vi "Check error type.vi"(8 "error in (no error)":errorcluster, 10 "Error cluster":T1={"jth object"="", "required object name"="", "Array element index"=0, "Element found?"=TRUE, "Array of clusters?"=FALSE, "key"="", "value"="", "key given?"=FALSE}, 11 "Datatype":T2) -> (0 "error out":errorcluster, 3 "Error string":string)   [LabVIEW 2015]
uses:
  Type Definitions/Basic datatypes.ctl
  Type Definitions/Error cluster.ctl
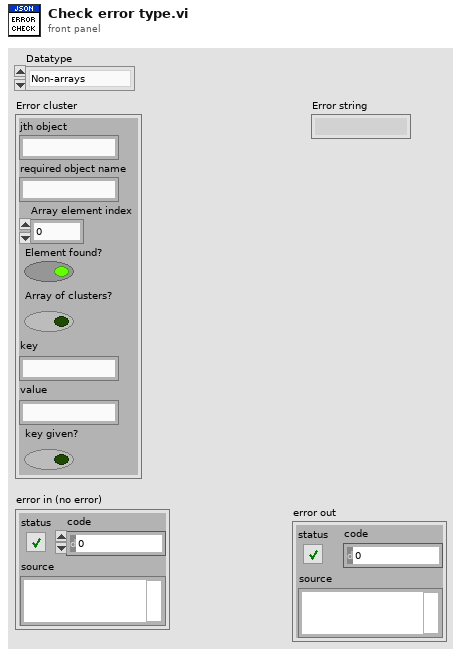
[diagram p1: front panel]
types:
  T1 = typedef "Error cluster.ctl" = cluster{"jth object":string, "required object name":string, "Array element index":u64, "Element found?":bool, "Array of clusters?":bool, "key":string, "value":string, "key given?":bool}
  T2 = typedef "Basic datatypes.ctl" = enum16{"Non-arrays", "Non-indexed array", "Indexed array"}
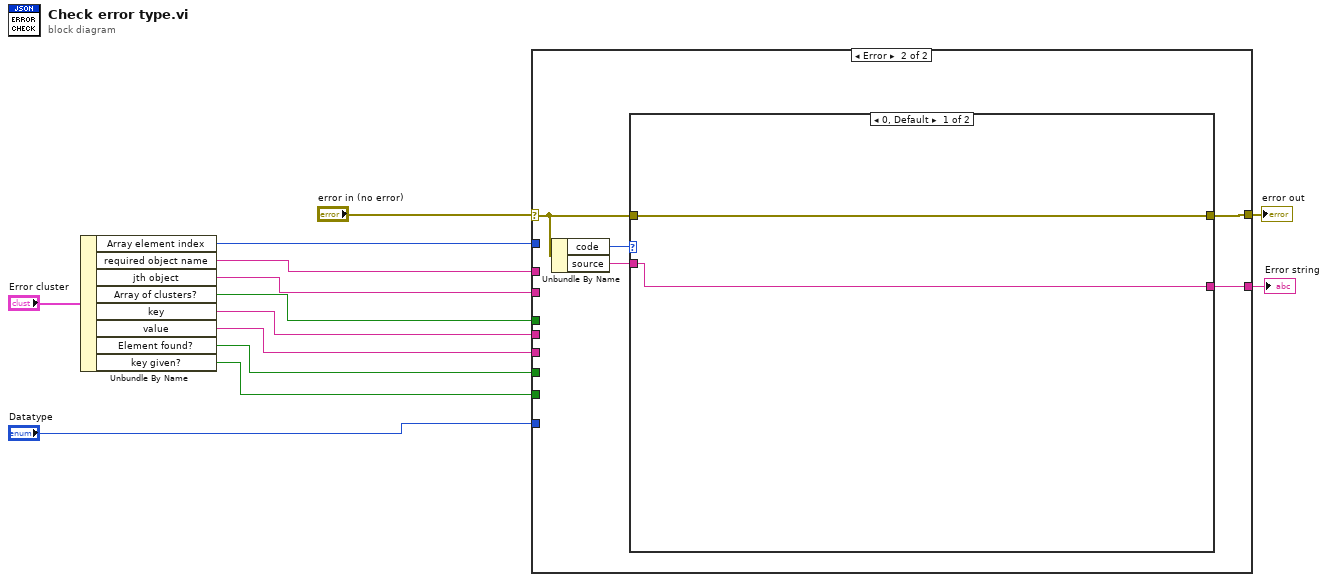
[diagram p0: block diagram]
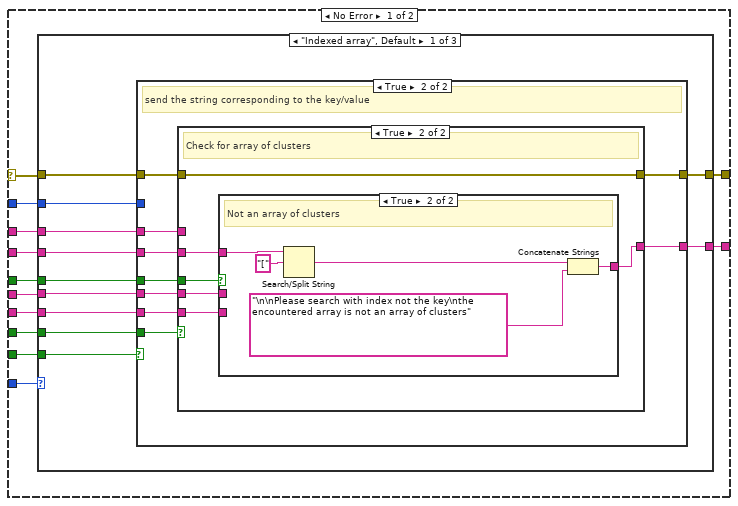
[diagram p2: hidden frame]
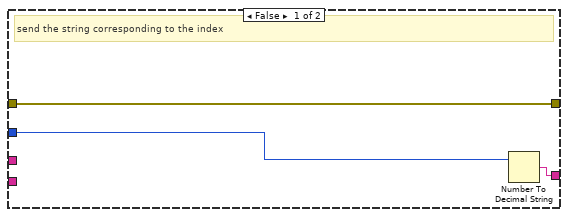
[diagram p3: hidden frame]
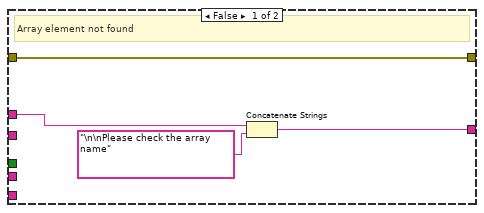
[diagram p4: hidden frame]
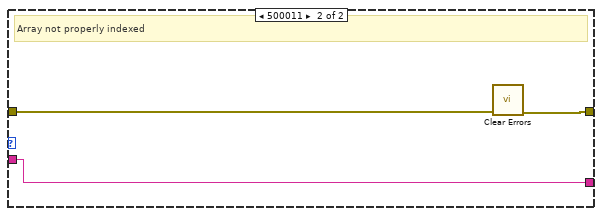
[diagram p8: hidden frame]
diagram:
  n1 = Unbundle By Name("Error cluster") -> ("Array element index"=w9:u64, "required object name"=w8:string, "jth object"=w7:string, "Array of clusters?"=w6:bool, "key"=w5:string, "value"=w4:string, "Element found?"=w2:bool, "key given?"=w3:bool)
  n2 = case shown="Error" "error in (no error)" {
    selector: "error in (no error)" -> [w14 w71]
    tunnel: [w25 w69] -> w13
    tunnel: [w24 w72] -> w12
    tunnel: "Datatype" -> [w23 _]
    tunnel: w9 -> [w22 _]
    tunnel: w8 -> [w21 _]
    tunnel: w7 -> [w20 _]
    tunnel: w6 -> [w19 _]
    tunnel: w5 -> [w18 _]
    tunnel: w4 -> [w17 _]
    tunnel: w3 -> [w16 _]
    tunnel: w2 -> [w15 _]
    frame No Error {
      n3 = case shown="\"Indexed array\", Default" w23 {
        tunnel: w21 -> [w26 _ w68]
        tunnel: w17 -> [w36 _ _]
        tunnel: w22 -> [w35 _ _]
        tunnel: w16 -> [w34 _ _]
        tunnel: w18 -> [w33 _ _]
        tunnel: [w32 w66 w68] -> w25
        tunnel: w20 -> [w31 w66 _]
        tunnel: w14 -> [w30 w65 w67]
        tunnel: [w29 w65 w67] -> w24
        tunnel: w15 -> [w28 _ _]
        tunnel: w19 -> [w27 _ _]
        frame "Indexed array", Default {
          n4 = case shown="True" w34 {
            tunnel: w33 -> [_ w46]
            tunnel: [w38 w47] -> w32
            tunnel: w35 -> [w39 _]
            tunnel: w36 -> [_ w48]
            tunnel: w26 -> [_ w44]
            tunnel: w31 -> [_ w45]
            tunnel: w30 -> [w37 w42]
            tunnel: [w37 w43] -> w29
            tunnel: w28 -> [_ w41]
            tunnel: w27 -> [_ w40]
            frame False {
              # "send the string corresponding to the index"
              n5 = Number To Decimal String(number=w39) -> (decimal integer string=w38:string)  [unwired: 1 in]
            }
            frame True {
              # "send the string corresponding to the key/value"
              n6 = case shown="True" w41 {
                tunnel: w48 -> [_ w58]
                tunnel: [w50 w57] -> w47
                tunnel: w46 -> [_ w56]
                tunnel: w45 -> [_ w55]
                tunnel: w44 -> [w52 _]
                tunnel: w42 -> [w49 w54]
                tunnel: [w49 w54] -> w43
                tunnel: w40 -> [_ w53]
                frame False {
                  # "Array element not found"
                  n7 = Concatenate Strings(w52, "\n\nPlease check the array name" ("string")) -> (w50:string)
                }
                frame True {
                  # "Check for array of clusters"
                  n8 = case shown="True" w53 {
                    tunnel: w58 -> [_ _]
                    tunnel: [w59 w60] -> w57
                    tunnel: w56 -> [w59 _]
                    tunnel: w55 -> [_ w63]
                    frame False {
                      # "cluster error (ele not found inside cluster)"
                    }
                    frame True {
                      # "Not an array of clusters"
                      n9 = Search/Split String(string=w63, search string/char (-)="[") -> (match + rest of string=w62:string)  [unwired: 1 in, 2 out]
                      n10 = Concatenate Strings(w62, "\n\nPlease search with index not the key\nthe encountered array is not an array of clusters" ("value")) -> (w60:string)
                    }
                  }
                }
              }
            }
          }
        }
        frame "Non-arrays" {
        }
        frame "Non-indexed array" {
          # "send the object name if empty braces[] are encountered"
        }
      }
    }
    frame Error {
      n11 = Unbundle By Name(w71) -> ("code"=w73:i32, "source"=w70:string)
      n12 = case shown="0, Default" w73 {
        tunnel: [w74 w77] -> w72
        tunnel: w71 -> [w74 w78]
        tunnel: w70 -> [w75 w76]
        tunnel: [w75 w76] -> w69
        frame 0, Default {
        }
        frame 500011 {
          # "Array not properly indexed"
          n13 = call <vilib>:"Clear Errors.vi"("error in (no error)"=w78) -> ("error out"=w77:errorcluster)  [unwired: 5 in, 1 out]
        }
      }
    }
  }
  "Error string" <- w13
  "error out" <- w12
